vi "BasicExampleOCP.vi"() -> ()   [LabVIEW 2020]
uses:
  PalmSens/PalmSens.lvclass
  D:/PalmSensAppsAndSDKS/LabVIEW/PalmSens SDK for LabVIEW 5.10/PalmSens/Libraries/PalmSens.Core.dll
  PalmSens/Libraries/PalmSens.Core.dll
  PalmSens/LiveCurveResult.ctl
  PalmSens/MeasurementResults.ctl
  PalmSens/MeasurementsResult.ctl
panel:
  out "Method .NET Refnum":refnum<k24>
  out "Measurements":T1
  out "Array":string[](array[string])
  out "Is Measuring":bool
  in  "PalmSens.lvclass":refnum<class "PalmSens.lvclass">
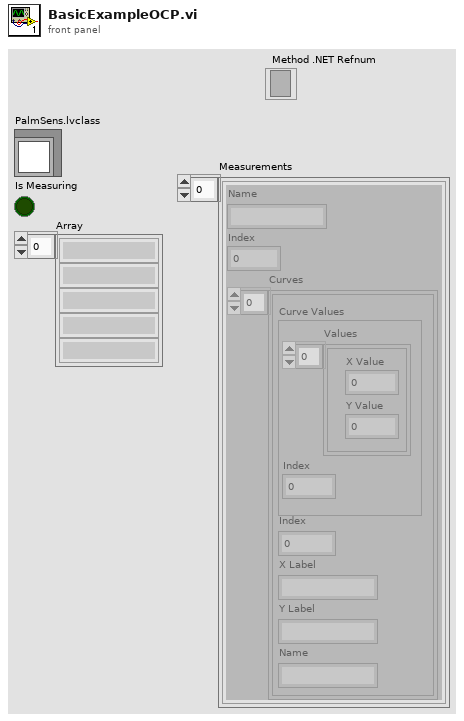
[diagram p1: front panel]
types:
  T1 = typedef "MeasurementsResult.ctl" = cluster{"Name":string, "Curves":T2, "Index":i32}[]
  T2 = typedef "MeasurementResults.ctl" = T3[]
  T3 = typedef "LiveCurveResult.ctl" = cluster{"X Label":string, "Y Label":string, "Name":string, "Index":i16, "Curve Values":cluster{"Values":cluster{"X Value":dbl, "Y Value":dbl}[], "Index":i16}}
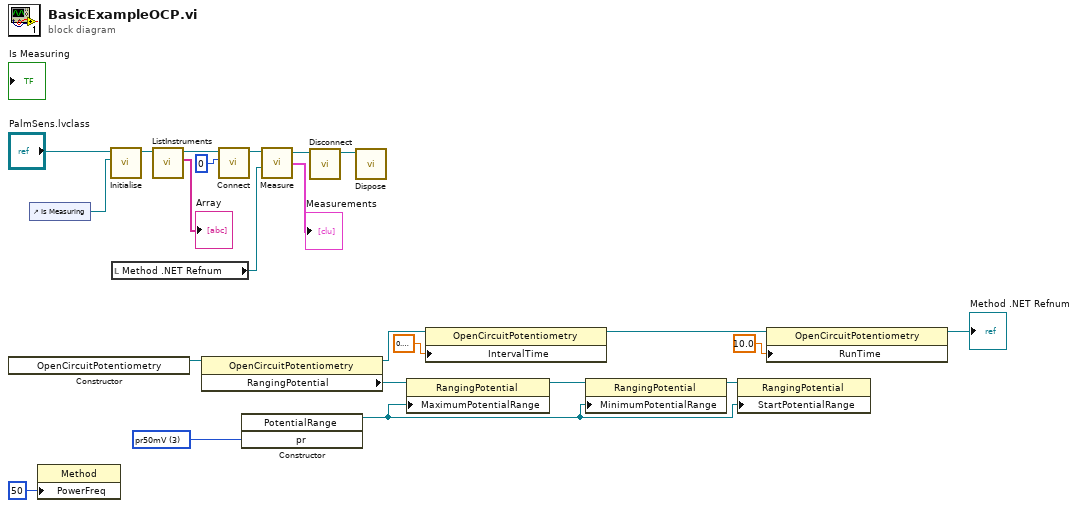
[diagram p0: block diagram]
diagram:
  w10 = 3 items=["pr1mV", "pr10mV", "pr20mV", "pr50mV", "pr100mV", "pr200mV", "pr500mV", "pr1V"] ("pr")
  n1 = constructor class="OpenCircuitPotentiometry"() -> (reference out=w12:refnum<k24>)  [unwired: 3 in, 2 out]
  n2 = control-ref of="Is Measuring"() -> (w22:refnum<vi>)
  n3 = property class="Method"("PowerFreq"=50) -> ()  [unwired: 2 in, 2 out]
  n4 = call-dynamic "Initialise.vi"("Is Measuring Refnum"=w22, "PalmSens in"="PalmSens.lvclass") -> ("PalmSens out"=w21:refnum<class "PalmSens.lvclass">)  [unwired: 8 in, 1 out]
  n5 = local read "Method .NET Refnum"() -> (w1:refnum<k24>)
  n6 = call-dynamic "ListInstruments.vi"("PalmSens in"=w21) -> ("Array"=→"Array":string[], "PalmSens out"=w19:refnum<class "PalmSens.lvclass">)  [unwired: 8 in, 1 out]
  n7 = property class="OpenCircuitPotentiometry"(reference=w12) -> (reference out=w5:refnum<k24>, "RangingPotential"=w11:refnum<k24>)  [unwired: 1 in, 1 out]
  n8 = call-dynamic "Connect.vi"("Instrument Index"=0, "PalmSens in"=w19) -> ("PalmSens out"=w16:refnum<class "PalmSens.lvclass">)  [unwired: 8 in, 1 out]
  n9 = constructor class="PotentialRange"("pr"=w10) -> (reference out=w7:refnum<k24>)  [unwired: 3 in, 3 out]
  n10 = call-dynamic "Measure.vi"("Method .NET Refnum"=w1, "PalmSens in"=w16) -> ("Curves"=→"Measurements":T2, "PalmSens out"=w14:refnum<class "PalmSens.lvclass">)  [unwired: 2 in, 1 out]
  n11 = call-dynamic "Disconnect.vi"("PalmSens in"=w14) -> ("PalmSens out"=w13:refnum<class "PalmSens.lvclass">)  [unwired: 9 in, 1 out]
  n12 = call-dynamic "Dispose.vi"("PalmSens in"=w13) -> ()  [unwired: 9 in, 2 out]
  n13 = property class="RangingPotential"(reference=w11, "MaximumPotentialRange"=w7) -> (reference out=w9:refnum<k24>)  [unwired: 1 in, 1 out]
  n14 = property class="OpenCircuitPotentiometry"(reference=w5, "IntervalTime"=sgl 0.1) -> (reference out=w4:refnum<k24>)  [unwired: 1 in, 1 out]
  n15 = property class="RangingPotential"(reference=w9, "MinimumPotentialRange"=w7) -> (reference out=w8:refnum<k24>)  [unwired: 1 in, 1 out]
  n16 = property class="RangingPotential"(reference=w8, "StartPotentialRange"=w7) -> ()  [unwired: 1 in, 2 out]
  n17 = property class="OpenCircuitPotentiometry"(reference=w4, "RunTime"=sgl 10.0) -> (reference out=→"Method .NET Refnum":refnum<k24>)  [unwired: 1 in, 1 out]
